vi "IPv4-Create.vi"(8 "Protocol":u8, 9 "Source IP":u8[](array[numeric])=[192, 168, 1, 200], 10 "Destination IP":u8[](array[numeric])=[192, 168, 1, 201], 11 "IPv4\nPayload":u8[](array[numeric])=[8, 0, 77, 77, 0, 1, 0, 14, 97, 98, 99, 100, 101, 102, 103, 104, 105, 106, 107, 108, 109, 110, 111, 112, 113, 114, 115, 116, 117, 118, 119, 97, 98, 99, 100, 101, 102, 103, 104, 105] format="%02x") -> (3 "IPv4 Packet":u8[](array[numeric]) format="%02x")   [LabVIEW 2018]
uses:
  Tests/FPGANic/FPGANic.Globals.vi
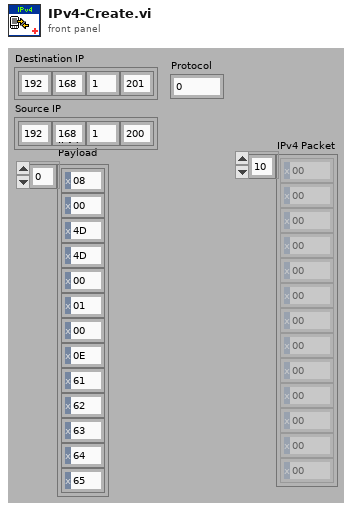
[diagram p1: front panel]
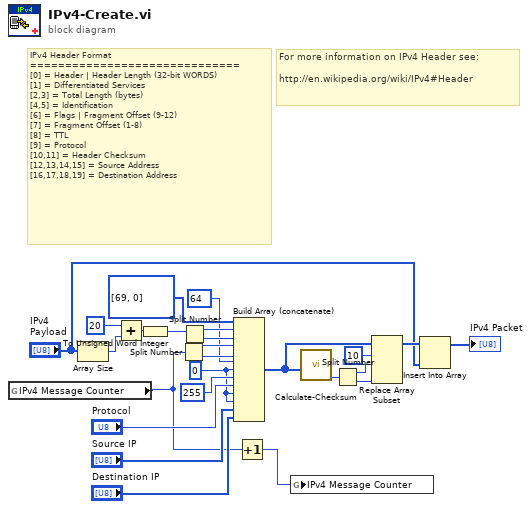
[diagram p0: block diagram]
diagram:
  w14 = u8 0 ("element")
  # "IPv4 Header Format\n==============================\n[0] = Header | Header Length (32-bit WORDS)\n[1] = Differentiated Services\n[2,3] = Total Length (bytes)\n[4,5] = Identification\n[6] = Flags | Fragment Offset (9-12)\n[7] = Fragment Offset (1-8)\n[8] = TTL\n[9] = Protocol\n[10,11] = Header Checksum\n[12,13,14,15] = Source Address\n[16,17,18,19] = Destination Address"
  # "For more information on IPv4 Header see:\n\nhttp://en.wikipedia.org/wiki/IPv4#Header"
  n1 = global read "FPGANic.Globals.vi" "IPv4 Message Counter"() -> (w1:i16)
  n2 = Array Size(array="IPv4\nPayload") -> (size(s)=w25:i32)
  n3 = Add(x=20, y=w25) -> (x+y=w22:i32)
  n4 = To Unsigned Word Integer(number=w22) -> (unsigned 16bit integer=w21:u16)
  n5 = Split Number(x=w1) -> (hi(x)=w18:u8, lo(x)=w17:u8)
  n6 = Split Number(x=w21) -> (hi(x)=w20:u8, lo(x)=w19:u8)
  n7 = Build Array (concatenate)(u8[] [69, 0], w20, w19, w18, w17, u8 64 ("element"), w14, u8 255 ("element"), "Protocol", w14, w14, "Source IP", "Destination IP") -> (w11:u8[])
  n8 = Increment(x=w1) -> (x+1=w2:i16)
  n9 = global write "FPGANic.Globals.vi" "IPv4 Message Counter"(w2) -> ()
  n10 = call "Calculate-Checksum.vi"("Array"=w11) -> ("Checksum"=w9:u16)  [unwired: 9 in, 1 out]
  n11 = Split Number(x=w9) -> (hi(x)=w8:u8, lo(x)=w7:u8)
  n12 = Replace Array Subset(array=w11, new element #1=w8, index #1=10 ("index"), new element #2=w7) -> (w6:u8[])  [unwired: 1 in]
  n13 = Insert Into Array(array=w6, new element="IPv4\nPayload") -> (→"IPv4 Packet":u8[])  [unwired: 1 in]
